vi "FT10_M4X Read.vi"(11 "Message Handling Cluster in":T1) -> (1 "Waveform Array":waveform(dbl)[](graph), 2 "Analysis Cluster Array":T12(array[cluster]), 3 "Message Handling Cluster out":T1)   [LabVIEW 2015]
uses:
  Controls/Control_Message Handling Cluster.ctl
  Controls/Control_M4X Connection.ctl
  Controls/Control_PXI-7854R FPGA Reference.ctl
  Controls/Control_Config Cluster.ctl
  Controls/Control_Config Unitherm Port.ctl
  Controls/Control_Config Simulate Values.ctl
  Controls/Control_Log Queue.ctl
  Controls/Control_Log Cluster.ctl
  Controls/Control_Log Time.ctl
  Controls/Control_Log Waveform Cluster.ctl
  Controls/Control_Log Analysis Cluster.ctl
  Controls/Control_Log Flag.ctl
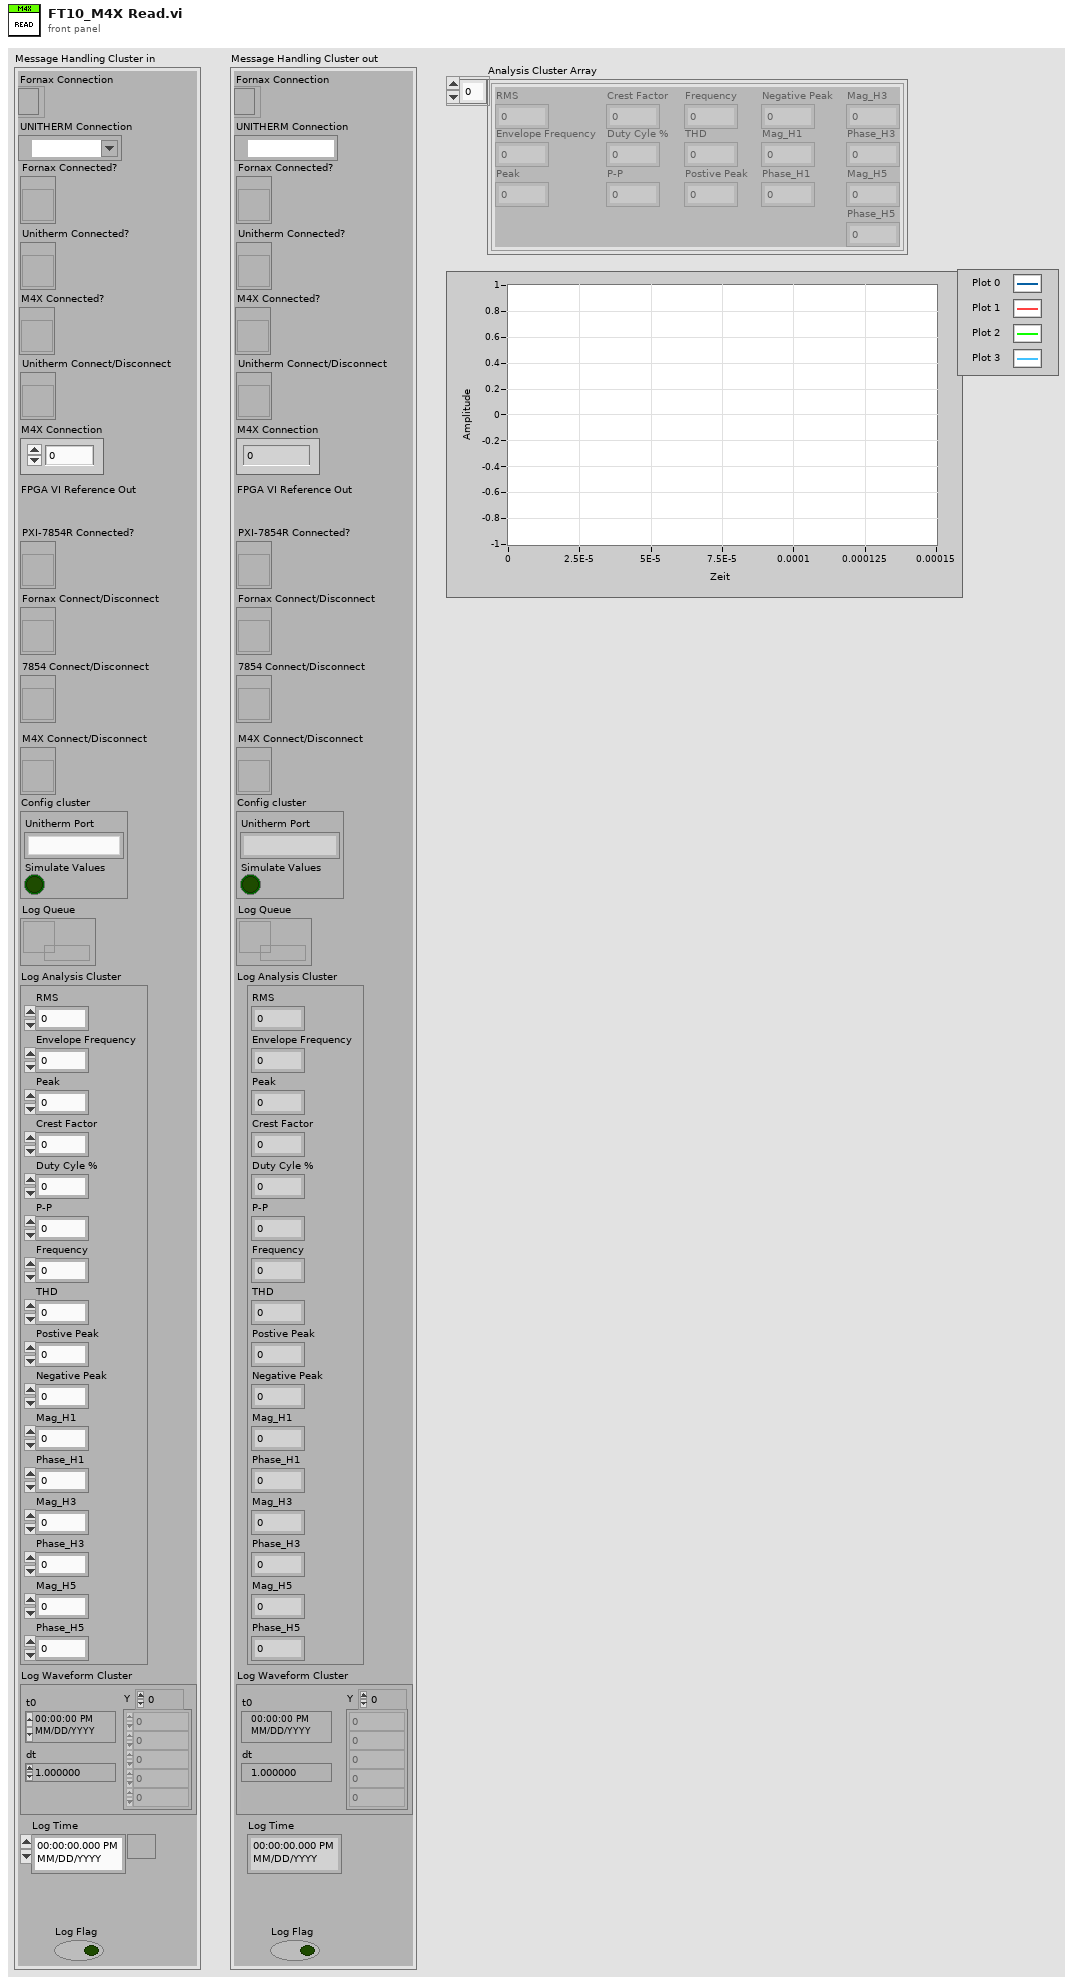
[diagram p1: front panel]
types:
  T1 = typedef "Control_Message Handling Cluster.ctl" = cluster{"Fornax Connected?":refnum<vi>, "Unitherm Connected?":refnum<vi>, "M4X Connected?":refnum<vi>, "Unitherm Connect/Disconnect":refnum<vi>, "Fornax Connection":refnum<k5>, "UNITHERM Connection":refnum<visa-resource-name>, "M4X Connection":T2, "PXI-7854R FPGA Reference":T3, "PXI-7854R Connected?":refnum<vi>, "Fornax Connect/Disconnect":refnum<vi>, "7854 Connect/Disconnect":refnum<vi>, "M4X Connect/Disconnect":refnum<vi>, "Config Cluster":T4, "Log Queue":T7, "Log Analysis Cluster":T8, "Log Waveform Cluster":T9, "Log Time":T10, "Log Flag":T11}
  T2 = typedef "Control_M4X Connection.ctl" = u32
  T3 = typedef "Control_PXI-7854R FPGA Reference.ctl" = refnum<k20>
  T4 = typedef "Control_Config Cluster.ctl" = cluster{"Unitherm Port":T5, "Simulate Values":T6}
  T5 = typedef "Control_Config Unitherm Port.ctl" = string
  T6 = typedef "Control_Config Simulate Values.ctl" = bool
  T7 = typedef "Control_Log Queue.ctl" = refnum<queue>
  T8 = typedef "Control_Log Analysis Cluster.ctl" = cluster{"RMS":dbl, "Envelope Frequency":dbl, "Peak":dbl, "Crest Factor":dbl, "Duty Cyle %":dbl, "P-P":dbl, "Frequency":dbl, "THD":dbl, "Postive Peak":dbl, "Negative Peak":dbl, "Mag_H1":dbl, "Phase_H1":dbl, "Mag_H3":dbl, "Phase_H3":dbl, "Mag_H5":dbl, "Phase_H5":dbl}
  T9 = typedef "Control_Log Waveform Cluster.ctl" = waveform(dbl)
  T10 = typedef "Control_Log Time.ctl" = timestamp
  T11 = typedef "Control_Log Flag.ctl" = bool
  T12 = cluster{"RMS":dbl, "Envelope Frequency":dbl, "Peak":dbl, "Crest Factor":dbl, "Duty Cyle %":dbl, "P-P":dbl, "Frequency":dbl, "THD":dbl, "Postive Peak":dbl, "Negative Peak":dbl, "Mag_H1":dbl, "Phase_H1":dbl, "Mag_H3":dbl, "Phase_H3":dbl, "Mag_H5":dbl, "Phase_H5":dbl}[]
  T13 = cluster{"RMS":dbl, "Envelope Frequency":dbl, "Peak":dbl, "Crest Factor":dbl, "Duty Cyle %":dbl, "P-P":dbl, "Frequency":dbl, "THD":dbl, "Postive Peak":dbl, "Negative Peak":dbl, "Mag_H1":dbl, "Phase_H1":dbl, "Mag_H3":dbl, "Phase_H3":dbl, "Mag_H5":dbl, "Phase_H5":dbl}
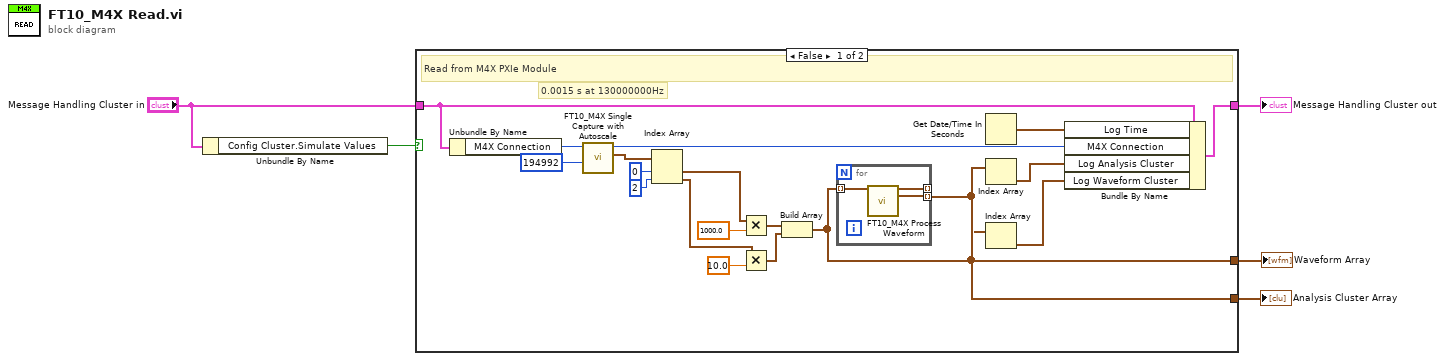
[diagram p0: block diagram]
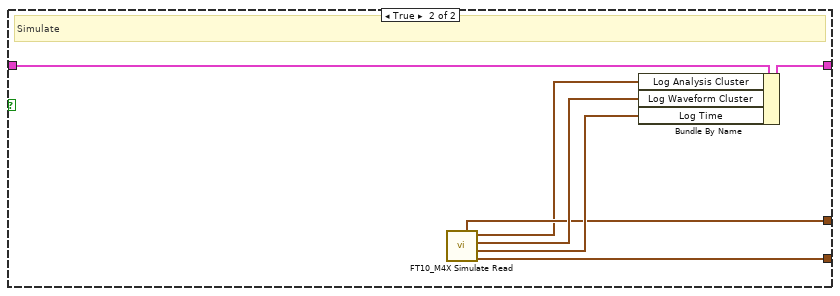
[diagram p2: hidden frame]
diagram:
  n1 = Unbundle By Name("Message Handling Cluster in") -> ("Config Cluster.Simulate Values"=w3:T6)
  n2 = case shown="False" w3 {
    tunnel: "Message Handling Cluster in" -> [w12 w34]
    tunnel: [w11 w33] -> w5
    tunnel: [w10 w28] -> w2
    tunnel: [w8 w30] -> w1
    frame False {
      # "0.0015 s at 130000000Hz"
      # "Read from M4X PXIe Module"
      n3 = Unbundle By Name(w12) -> ("M4X Connection"=w14:T2)
      n4 = call "FT10_M4X Single Capture with Autoscale.vi"("memsize"=194992, "Card Handle in"=w14) -> ("Data"=w18:waveform(sgl)[], "Card Handle out"=w13:u32)  [unwired: 8 in]
      n5 = Index Array(array=w18, index #1=0 ("index"), index #2=2 ("index")) -> (element #1=w23:waveform(sgl), element #2=w24:waveform(sgl))
      n6 = Multiply(x=w23, y=1000.0) -> (x*y=w21:waveform(dbl))
      n7 = Multiply(x=w24, y=10.0) -> (x*y=w22:waveform(dbl))
      n8 = Build Array(w21, w22) -> (w8:waveform(dbl)[])
      n9 = for {
        tunnel: w8 -> [w25] mode=indexing
        tunnel: [w27] -> w10 mode=indexing
        tunnel: [w26] -> _ mode=indexing
        n10 = call "FT10_M4X Process Waveform.vi"("RF Waveform In"=w25) -> ("RF Waveform Out"=w26:waveform(sgl), "Measurements"=w27:T13)  [unwired: 12 in, 1 out]
      }
      n11 = Get Date/Time In Seconds() -> (seconds since 1Jan1904=w6:timestamp)
      n12 = Index Array(array=w10) -> (element=w9:T13)  [unwired: 1 in]
      n13 = Index Array(array=w8) -> (element=w7:waveform(dbl))  [unwired: 1 in]
      n14 = Bundle By Name(cluster=w12, "Log Time"=w6, "M4X Connection"=w13, "Log Analysis Cluster"=w9, "Log Waveform Cluster"=w7) -> (w11:T1)
    }
    frame True {
      # "Simulate"
      n15 = call "FT10_M4X Simulate Read.vi"() -> ("Analysis Cluster Array"=w28:T8[], "seconds since 1Jan1904"=w32:timestamp, "Log Waveform Cluster"=w31:T9, "Simulated Log Analysis Cluster"=w29:T8, "Simulated Waveform Array"=w30:T9[])  [unwired: 7 in]
      n16 = Bundle By Name(cluster=w34, "Log Analysis Cluster"=w29, "Log Waveform Cluster"=w31, "Log Time"=w32) -> (w33:T1)
    }
  }
  "Message Handling Cluster out" <- w5
  "Waveform Array" <- w1
  "Analysis Cluster Array" <- w2
